vi "OperaçõesVariáveis.vi"(3 "Entradas":T2, 4 "Escrever?":bool, 5 "NXT IN":T4) -> (0 "Mensagens":T3, 1 "Saídas":T1, 2 "NXT OUT":T4)   [LabVIEW 2012, in "ExemploFinal.lvrbt"]
uses:
  ExemploFinal.lvrbt
  <vilib>/NXT/Subs/LVHSConnector.ctl
  <vilib>/NXT/LegoClasses/BrickReference/BrickReference.lvclass
  <vilib>/NXT/Dual Mode Library/Advanced/NXTFlag_Get.vi
  <vilib>/NXT/Dual Mode Library/Advanced/NXTFlag_Get_Integer.vi
  <vilib>/NXT/Dual Mode Library/Advanced/NXTFlag_Get_String.vi
  <vilib>/NXT/Dual Mode Library/Advanced/NXTFlag_Assign.vi
  <vilib>/NXT/Dual Mode Library/Advanced/NXTFlag_Assign_String.vi
  <vilib>/NXT/Dual Mode Library/Advanced/NXTFlag_Assign_integer.vi
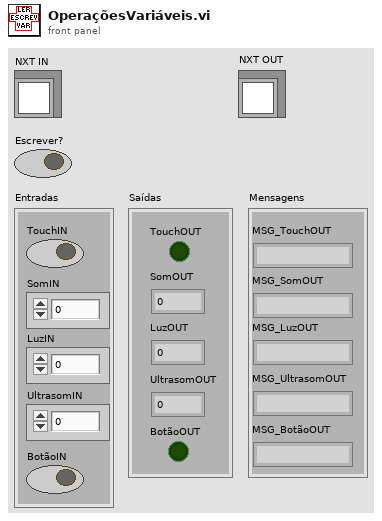
[diagram p1: front panel]
types:
  T1 = cluster{"TouchOUT":bool, "SomOUT":i32, "LuzOUT":i32, "UltrasomOUT":i32, "BotãoOUT":bool}
  T2 = cluster{"TouchIN":bool, "SomIN":i16, "LuzIN":i16, "UltrasomIN":i16, "BotãoIN":bool}
  T3 = cluster{"MSG_TouchOUT":string, "MSG_SomOUT":string, "MSG_LuzOUT":string, "MSG_UltrasomOUT":string, "MSG_BotãoOUT":string}
  T4 = typedef "LVHSConnector.ctl" = refnum<class "BrickReference.lvclass">
  T5 = cluster{"BotãoOUT":bool, "UltrasomOUT":i32, "LuzOUT":i32, "SomOUT":i32, "TouchOUT":bool}
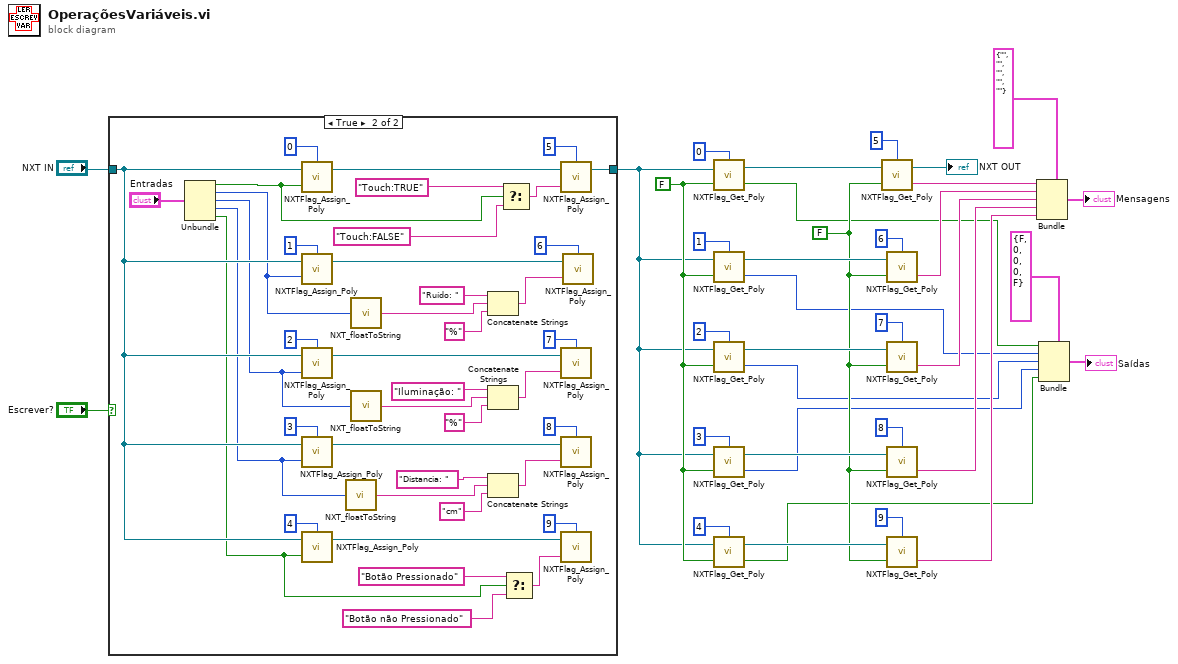
[diagram p0: block diagram]
diagram:
  w16 = FALSE ("Clear if Found")
  w32 = FALSE ("Clear if Found")
  n1 = case shown="True" "Escrever?" {
    tunnel: "NXT IN" -> [w36 w44]
    tunnel: [w36 w43] -> w31
    frame False {
    }
    frame True {
      n2 = Unbundle("Entradas") -> ("TouchIN"=w41:bool, "SomIN"=w40:i16, "LuzIN"=w39:i16, "UltrasomIN"=w38:i16, "BotãoIN"=w37:bool)
      n3 = call-poly <vilib>:"NXTFlag_Assign_Poly.vi"("Flag State"=w41, "NXT/EV3"=w44, "NXT/EV3 Flag Number"=i8 0) -> ("NXT/EV3"=w67:T4)  [unwired: 1 in]
      n4 = call-poly <vilib>:"NXTFlag_Assign_Poly.vi"("Flag Value"=w40, "NXT/EV3"=w44, "NXT/EV3 Flag Number"=i8 1) -> ("NXT/EV3"=w66:T4)  [unwired: 1 in]
      n5 = call-poly <vilib>:"NXTFlag_Assign_Poly.vi"("Flag Value"=w39, "NXT/EV3"=w44, "NXT/EV3 Flag Number"=i8 2) -> ("NXT/EV3"=w65:T4)  [unwired: 1 in]
      n6 = call-poly <vilib>:"NXTFlag_Assign_Poly.vi"("Flag Value"=w38, "NXT/EV3"=w44, "NXT/EV3 Flag Number"=i8 3) -> ("NXT/EV3"=w64:T4)  [unwired: 1 in]
      n7 = call-poly <vilib>:"NXTFlag_Assign_Poly.vi"("Flag State"=w37, "NXT/EV3"=w44, "NXT/EV3 Flag Number"=i8 4) -> ("NXT/EV3"=w63:T4)  [unwired: 1 in]
      n8 = call <vilib>:"NXT_floatToString.vi"("number"=w38) -> ("string"=w52:string)
      n9 = call <vilib>:"NXT_floatToString.vi"("number"=w40) -> ("string"=w57:string)
      n10 = call <vilib>:"NXT_floatToString.vi"("number"=w39) -> ("string"=w56:string)
      n11 = Concatenate Strings("Ruído: ", w57, "%") -> (w58:string)
      n12 = Concatenate Strings("Iluminação: ", w56, "%") -> (w54:string)
      n13 = Concatenate Strings("Distancia: ", w52, "cm") -> (w51:string)
      n14 = Select(t="Touch:TRUE", s=w41, f="Touch:FALSE") -> (s? t:f=w62:string)
      n15 = Select(t="Botão Pressionado", s=w37, f="Botão não Pressionado") -> (s? t:f=w48:string)
      n16 = call-poly <vilib>:"NXTFlag_Assign_Poly.vi"("Flag Value"=w62, "NXT/EV3"=w67, "NXT/EV3 Flag Number"=i8 5) -> ("NXT/EV3"=w43:T4)  [unwired: 1 in]
      n17 = call-poly <vilib>:"NXTFlag_Assign_Poly.vi"("Flag Value"=w54, "NXT/EV3"=w65, "NXT/EV3 Flag Number"=i8 7) -> ()  [unwired: 1 in, 1 out]
      n18 = call-poly <vilib>:"NXTFlag_Assign_Poly.vi"("Flag Value"=w51, "NXT/EV3"=w64, "NXT/EV3 Flag Number"=i8 8) -> ()  [unwired: 1 in, 1 out]
      n19 = call-poly <vilib>:"NXTFlag_Assign_Poly.vi"("Flag Value"=w48, "NXT/EV3"=w63, "NXT/EV3 Flag Number"=i8 9) -> ()  [unwired: 1 in, 1 out]
      n20 = call-poly <vilib>:"NXTFlag_Assign_Poly.vi"("Flag Value"=w58, "NXT/EV3"=w66, "NXT/EV3 Flag Number"=i8 6) -> ()  [unwired: 1 in, 1 out]
    }
  }
  n21 = call-poly <vilib>:"NXTFlag_Get_Poly.vi"("Clear if Found"=w32, "NXT/EV3"=w31, "NXT/EV3 Flag Number"=0) -> ("status"=w1:bool, "NXT/EV3"=w26:T4)
  n22 = call-poly <vilib>:"NXTFlag_Get_Poly.vi"("Clear if Found"=w32, "NXT/EV3"=w31, "NXT/EV3 Flag Number"=1) -> ("Flag Value"=w2:i32, "NXT/EV3"=w23:T4)
  n23 = call-poly <vilib>:"NXTFlag_Get_Poly.vi"("Clear if Found"=w32, "NXT/EV3"=w31, "NXT/EV3 Flag Number"=2) -> ("Flag Value"=w3:i32, "NXT/EV3"=w21:T4)
  n24 = call-poly <vilib>:"NXTFlag_Get_Poly.vi"("Clear if Found"=w32, "NXT/EV3"=w31, "NXT/EV3 Flag Number"=3) -> ("Flag Value"=w4:i32, "NXT/EV3"=w18:T4)
  n25 = call-poly <vilib>:"NXTFlag_Get_Poly.vi"("Clear if Found"=w32, "NXT/EV3"=w31, "NXT/EV3 Flag Number"=4) -> ("status"=w5:bool, "NXT/EV3"=w17:T4)
  n26 = call-poly <vilib>:"NXTFlag_Get_Poly.vi"("Clear if Found"=w16, "NXT/EV3"=w26, "NXT/EV3 Flag Number"=5) -> ("Flag Value"=w12:string, "NXT/EV3"=→"NXT OUT":T4)
  n27 = call-poly <vilib>:"NXTFlag_Get_Poly.vi"("Clear if Found"=w16, "NXT/EV3"=w23, "NXT/EV3 Flag Number"=6) -> ("Flag Value"=w9:string)  [unwired: 1 out]
  n28 = call-poly <vilib>:"NXTFlag_Get_Poly.vi"("Clear if Found"=w16, "NXT/EV3"=w21, "NXT/EV3 Flag Number"=7) -> ("Flag Value"=w8:string)  [unwired: 1 out]
  n29 = call-poly <vilib>:"NXTFlag_Get_Poly.vi"("Clear if Found"=w16, "NXT/EV3"=w18, "NXT/EV3 Flag Number"=8) -> ("Flag Value"=w7:string)  [unwired: 1 out]
  n30 = call-poly <vilib>:"NXTFlag_Get_Poly.vi"("Clear if Found"=w16, "NXT/EV3"=w17, "NXT/EV3 Flag Number"=9) -> ("Flag Value"=w6:string)  [unwired: 1 out]
  n31 = Bundle(cluster=T3 {"MSG_TouchOUT"="", "MSG_SomOUT"="", "MSG_LuzOUT"="", "MSG_UltrasomOUT"="", "MSG_BotãoOUT"=""} ("Mensagens"), "MSG_TouchOUT"=w12, "MSG_SomOUT"=w9, "MSG_LuzOUT"=w8, "MSG_UltrasomOUT"=w7, "MSG_BotãoOUT"=w6) -> (→"Mensagens":T3)
  n32 = Bundle(cluster=T5 {"BotãoOUT"=FALSE, "UltrasomOUT"=0, "LuzOUT"=0, "SomOUT"=0, "TouchOUT"=FALSE} ("Saídas"), "BotãoOUT"=w1, "UltrasomOUT"=w2, "LuzOUT"=w3, "SomOUT"=w4, "TouchOUT"=w5) -> (→"Saídas":T5)
